vi "manage Buffer_Scope.vi"(1 "Cluster":cluster{"Diode":dbl, "Double Diode":dbl}, 2 "Buffer in":cluster{"Diode":dbl, "Double Diode":dbl}[](array[cluster]), 3 "Main Index":i32, 4 "Analysis Buffersize":i32) -> (5 "Buffer out":cluster{"Diode":dbl, "Double Diode":dbl}[](array[cluster]))   [LabVIEW 2009]
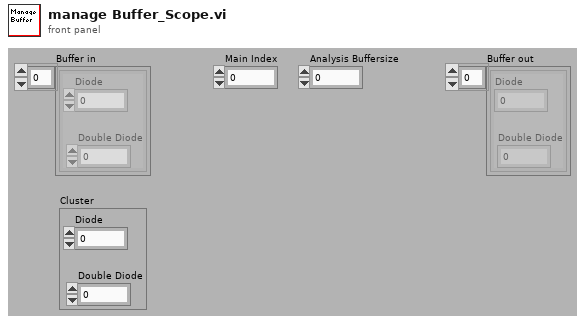
[diagram p1: front panel]
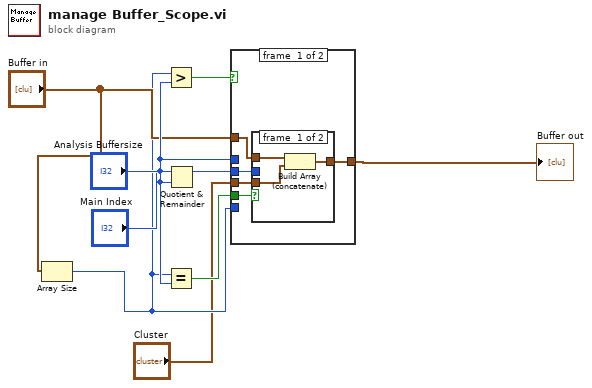
[diagram p0: block diagram]
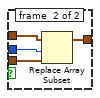
[diagram p2: hidden frame]
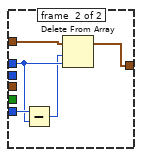
[diagram p3: hidden frame]
diagram:
  n1 = Array Size(array="Buffer in") -> (size(s)=w2:i32)
  n2 = Greater?(x=w2, y="Analysis Buffersize") -> (0:w4:bool)
  n3 = Equal?(x=w2, y="Analysis Buffersize") -> (x = y?=w9:bool)
  n4 = Quotient & Remainder(x="Main Index", y="Analysis Buffersize") -> (x-y*floor(x/y)=w6:i32)  [unwired: 1 out]
  n5 = case shown="False" w4 {
    tunnel: [w10 w22] -> w7
    tunnel: "Buffer in" -> [w11 w26]
    tunnel: "Analysis Buffersize" -> [_ w24]
    tunnel: w2 -> [_ w25]
    tunnel: "Cluster" -> [w12 _]
    tunnel: w6 -> [w13 _]
    tunnel: w9 -> [w14 _]
    frame #0 {
      n6 = case shown="True" w14 {
        tunnel: w13 -> [_ w21]
        tunnel: w12 -> [w16 w20]
        tunnel: w11 -> [w17 w19]
        tunnel: [w15 w18] -> w10
        frame #0 {
          n7 = Build Array (concatenate)(w17, w16) -> (w15:cluster{"Diode":dbl, "Double Diode":dbl}[])
        }
        frame #1 {
          n8 = Replace Array Subset(array=w19, new element=w20, index=w21) -> (w18:cluster{"Diode":dbl, "Double Diode":dbl}[])
        }
      }
    }
    frame #1 {
      n9 = Subtract(x=w25, y=w24) -> (x-y=w23:i32)
      n10 = Delete From Array(array=w26, length=w23, index=w24) -> (array with subset deleted=w22:cluster{"Diode":dbl, "Double Diode":dbl}[])  [unwired: 1 out]
    }
  }
  "Buffer out" <- w7
